vi "interp img path to lineout paths.vi"(8 "error in (no error)":errorcluster, 11 "Interp image path":path) -> (0 "error out":errorcluster, 2 "angle lineout path":path, 3 "Spectrum lineout path":path)   [LabVIEW 2013]
uses:
  Convert File Extension (Path)__ogtk.vi
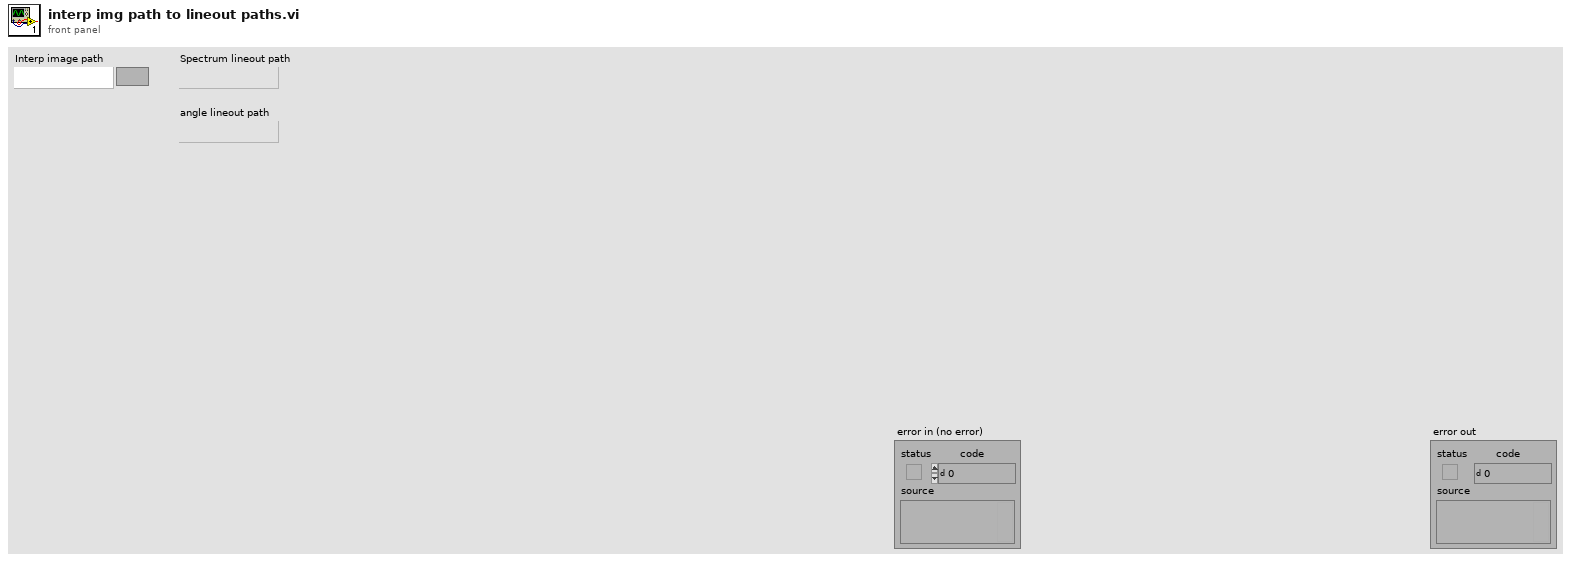
[diagram p1: front panel]
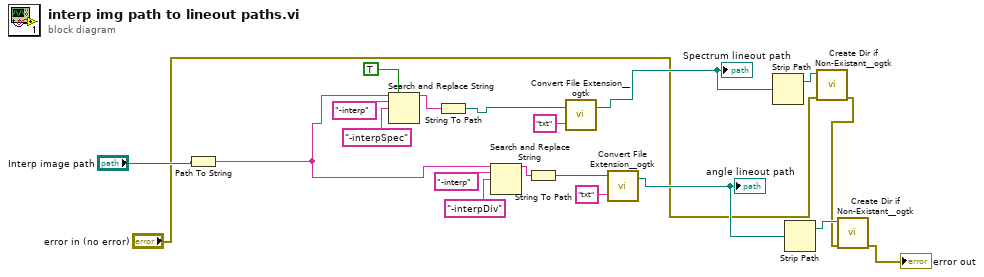
[diagram p0: block diagram]
diagram:
  n1 = Path To String(path="Interp image path") -> (string=w13:string)
  n2 = Search and Replace String(replace all?=TRUE ("replace all? (F)"), input string=w13, search string="-interp", replace string="-interpSpec") -> (result string=w11:string)  [unwired: 4 in, 3 out]
  n3 = String To Path(string=w11) -> (path=w8:path)
  n4 = Search and Replace String(input string=w13, search string="-interp", replace string="-interpDiv") -> (result string=w10:string)  [unwired: 5 in, 3 out]
  n5 = String To Path(string=w10) -> (path=w9:path)
  n6 = call-poly "Convert File Extension__ogtk.vi"("new ending (none)"="txt", "file name"=w8) -> ("new filename"=w6:path)  [unwired: 1 out]
  "Spectrum lineout path" <- w6
  n7 = call-poly "Convert File Extension__ogtk.vi"("new ending (none)"="txt", "file name"=w9) -> ("new filename"=w5:path)  [unwired: 1 out]
  "angle lineout path" <- w5
  n8 = Strip Path(path=w6) -> (stripped path=w7:path)  [unwired: 1 out]
  n9 = Strip Path(path=w5) -> (stripped path=w4:path)  [unwired: 1 out]
  n10 = call "Create Dir if Non-Existant__ogtk.vi"("error in (no error)"="error in (no error)", "Directory Path"=w7) -> ("error out"=w3:errorcluster)  [unwired: 7 in, 2 out]
  n11 = call "Create Dir if Non-Existant__ogtk.vi"("error in (no error)"=w3, "Directory Path"=w4) -> ("error out"=→"error out":errorcluster)  [unwired: 7 in, 2 out]
